vi "Handle Last Ack Core.vi"(4 "error in (no error)":errorcluster, 6 "Last Ack":refnum<class "Last Ack.lvclass">, 7 "Actor with Nesteds in":refnum<class "Actor with Nesteds.lvclass">) -> (0 "error out":errorcluster, 3 "Actor with Nesteds out":refnum<class "Actor with Nesteds.lvclass">)   [LabVIEW 2020, in "Nested Actor.lvlib" / "Actor with Nesteds.lvclass"]
doc: "<p>(<strong>Filename</strong>: <span class=\"dnl\">Actor Framework.lvlib:Actor.lvclass:Handle Last Ack Core.vi</span>)</p>\n<p>Defines how the caller actor responds to the Last Ack message from a nested actor. The Last Ack message is the final message a nested actor sends to its caller before it shuts down. The message contains information about the final state of the nested actor.</p>\n<p>By default, this method does nothing except return any error the nested actor sent. A descendant class may override this method to define behavior.</p>"
uses:
  Actor with Nesteds.lvclass
  Core/ActorFramework/LastAck/Last Ack.lvclass
  C:/Users/J63553/Projects/_LabVIEW Community/actor-framework/Core/ActorFramework/Actor/Actor.lvclass
  Core/ActorFramework/Message/Message.lvclass
  Core/ActorFramework/Actor/Actor.lvclass/Actor.ctl
  Core/ActorFramework/Message Enqueuer/Message Enqueuer.lvclass/Message Enqueuer.ctl
  Core/ActorFramework/Message Priority Queue/Priority Enqueue.vi
  Core/ActorFramework/Actor/Actor.lvclass
  Core/ActorFramework/Message Enqueuer/Message Enqueuer.lvclass
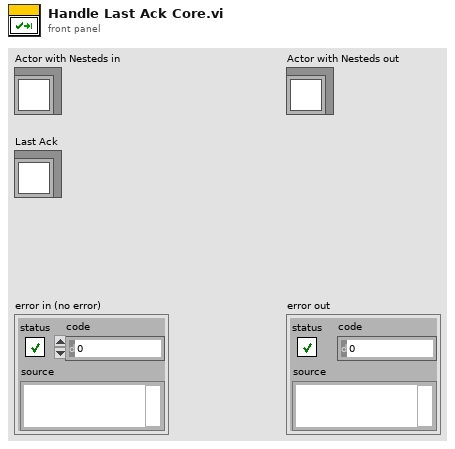
[diagram p1: front panel]
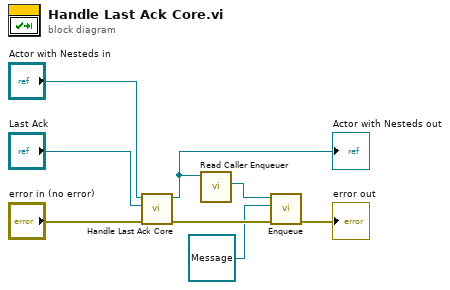
[diagram p0: block diagram]
diagram:
  n1 = call-parent "Handle Last Ack Core.vi"("error in (no error)"="error in (no error)", "Last Ack"="Last Ack", "Actor in"="Actor with Nesteds in") -> ("error out"=w8:errorcluster, "Actor out"=w3:refnum<class "Actor with Nesteds.lvclass">)  [unwired: 3 in]
  "Actor with Nesteds out" <- w3
  n2 = call "Read Caller Enqueuer.vi"("Actor"=w3) -> ("Caller Enqueuer"=w2:refnum<class "Message Enqueuer.lvclass">)  [unwired: 10 in]
  n3 = call "Enqueue.vi"("error in (no error)"=w8, "Message"=refnum<class "Message.lvclass"> refnum, "Message Enqueuer in"=w2) -> ("error out"=→"error out":errorcluster)  [unwired: 7 in, 1 out]
